vi "Error Query.vi"(8 "error in (no error)":errorcluster, 11 "VISA resource name":refnum<visa-resource-name>) -> (0 "error out":errorcluster, 1 "Error Message":string, 2 "Error Code":i32[](array[numeric]), 3 "VISA resource name out":refnum<visa-resource-name>)   [LabVIEW 2010, in "Keithley 24XX.lvlib"]
doc: "Queries the instrument for any errors in the instrument's error queue. It will continue to read errors until all errors have been read from the instrument. Any errors will be returned in the <B>error out</B> control.\n\nNote:\nThis VI is called automatically by most driver VIs so it is not usually necessary to call this in an application."
uses:
  <instrlib>/Keithley 24XX/Keithley 24XX.lvlib
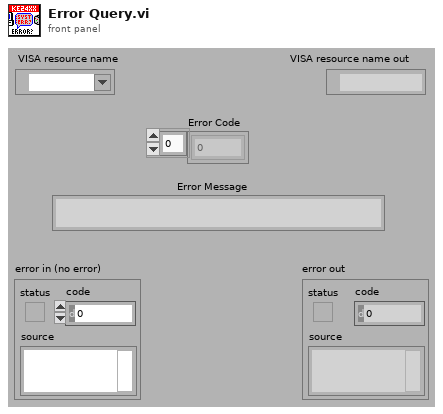
[diagram p1: front panel]
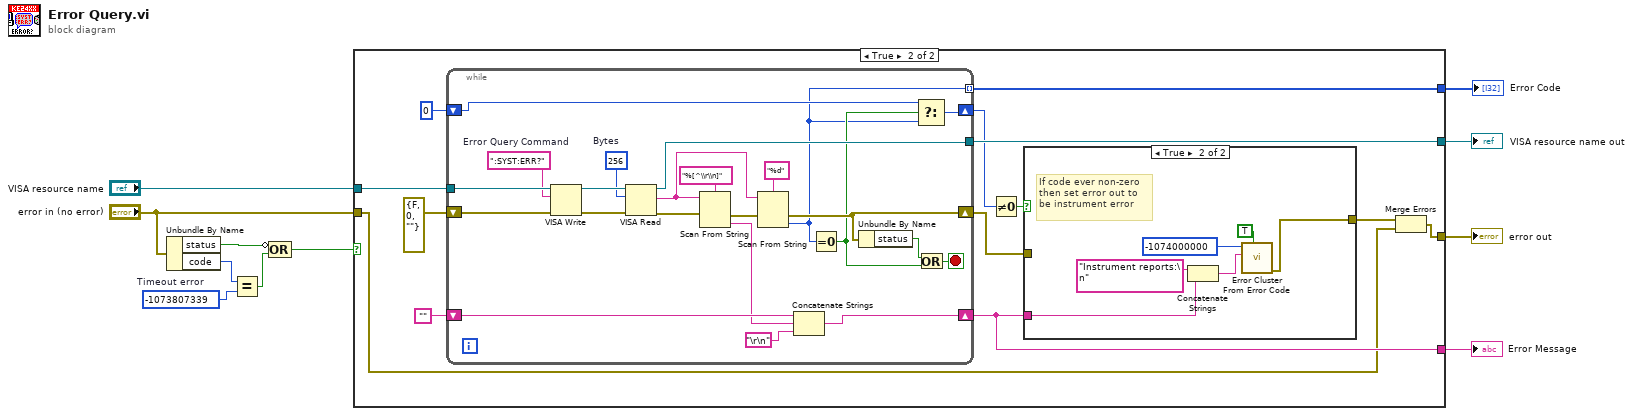
[diagram p0: block diagram]
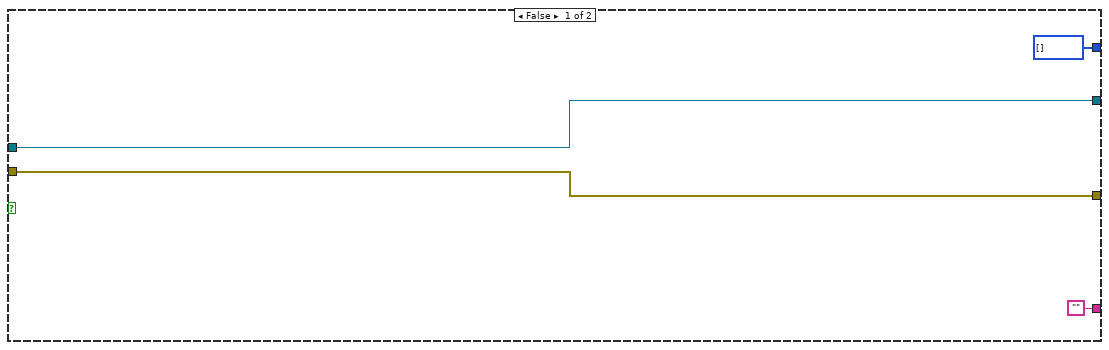
[diagram p2: hidden frame]
diagram:
  w6 = -1073807339  # Timeout error
  n1 = Unbundle By Name("error in (no error)") -> ("status"=w7:bool, "code"=w4:i32)
  n2 = Equal?(x=w4, y=w6) -> (x = y?=w5:bool)
  n3 = Compound Arithmetic op=OR(invert w7, w5) -> (w3:bool)
  n4 = case shown="True" w3 {
    tunnel: [w15 w28] -> w11
    tunnel: "VISA resource name" -> [w15 w27]
    tunnel: "error in (no error)" -> [w14 w17]
    tunnel: [w14 w25] -> w9
    tunnel: ["" w19] -> w2
    tunnel: [i32[] [] w18] -> w1
    frame False {
    }
    frame True {
      n5 = while {
        tunnel: [w58] -> w28
        tunnel: w27 -> [w57]
        shift-right: [w45] -> w19
        shift-left: "" -> [w48]
        shift-right: [w43] -> w20
        shift-left: 0 -> [w44]
        shift-right: [w41] -> w16
        shift-left: errorcluster {"status"=FALSE, "code"=0, "source"=""} ("error in (no error)") -> [w42]
        tunnel: [w36] -> w18 mode=indexing
        stop <- w51 stop-if-true
        w55 = u32 256  # Bytes
        w53 = ":SYST:ERR?"  # Error Query Command
        n6 = VISA Write(VISA resource name=w57, write buffer=w53, error in (no error)=w42) -> (VISA resource name out=w56:refnum<visa-resource-name>, error out=w54:errorcluster)  [unwired: 1 out]
        n7 = VISA Read(VISA resource name=w56, byte count=w55, error in (no error)=w54) -> (VISA resource name out=w58:refnum<visa-resource-name>, read buffer=w49:string, error out=w40:errorcluster)  [unwired: 1 out]
        n8 = Scan From String(format string="%[^\\r\\n]", input string=w49, error in=w40) -> (error out=w39:errorcluster, output 1=w46:string)  [unwired: 2 in, 2 out]
        n9 = Scan From String(format string="%d", input string=w49, error in=w39) -> (error out=w41:errorcluster, output 1=w36:i32)  [unwired: 2 in, 2 out]
        n10 = Concatenate Strings(w48, w46, "\r\n") -> (w45:string)
        n11 = Equal To 0?(x=w36) -> (x = 0?=w37:bool)
        n12 = Unbundle By Name(w41) -> ("status"=w38:bool)
        n13 = Select(t=w44, s=w37, f=w36) -> (s? t:f=w43:i32)
        n14 = Or(x=w38, y=w37) -> (x .or. y?=w51:bool)
      }
      n15 = Not Equal To 0?(x=w20) -> (x != 0?=w23:bool)
      n16 = case shown="True" w23 {
        tunnel: w19 -> [_ w34]
        tunnel: [w29 w30] -> w22
        tunnel: w16 -> [w29 _]
        frame False {
        }
        frame True {
          # "If code ever non-zero\nthen set error out to\nbe instrument error"
          n17 = Concatenate Strings("Instrument reports:\n" ("Source"), w34) -> (w31:string)
          n18 = call <vilib>:"Error Cluster From Error Code.vi"("show call chain? (False)"=TRUE, "error message (\"\")"=w31, "error code (0)"=-1074000000 ("Code")) -> ("error out"=w30:errorcluster)  [unwired: 6 in]
        }
      }
      n19 = Merge Errors(w22, w17) -> (w25:errorcluster)
    }
  }
  "VISA resource name out" <- w11
  "error out" <- w9
  "Error Message" <- w2
  "Error Code" <- w1
